vi "Calculate Timing Characteristics.vi"(10 "Engine Clock Rate (MHz)":i32=120000000 format="%.0p", 11 "SPI Signals":T2) -> (3 "Timing Characteristics":T1)   [LabVIEW 2014]
uses:
  Controls/Digital Data.ctl
  Controls/Timing Characteristics.ctl
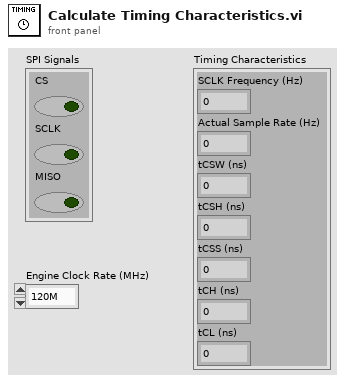
[diagram p1: front panel]
types:
  T1 = typedef "Timing Characteristics.ctl" = cluster{"SCLK Frequency (Hz)":dbl, "Actual Sample Rate (Hz)":dbl, "tCSW (ns)":dbl, "tCSH (ns)":dbl, "tCSS (ns)":dbl, "tCH (ns)":dbl, "tCL (ns)":dbl}
  T2 = typedef "Digital Data.ctl" = cluster{"CS":bool, "SCLK":bool, "MISO":bool}
  T3 = enum16{"A Rising, A Rising", "A Rising, A Falling", "A Falling, A Rising", "A Falling, A Falling", "A Rising, B Rising", "A Rising, B Falling", "A Falling, B Rising", "A Falling, B Falling"}
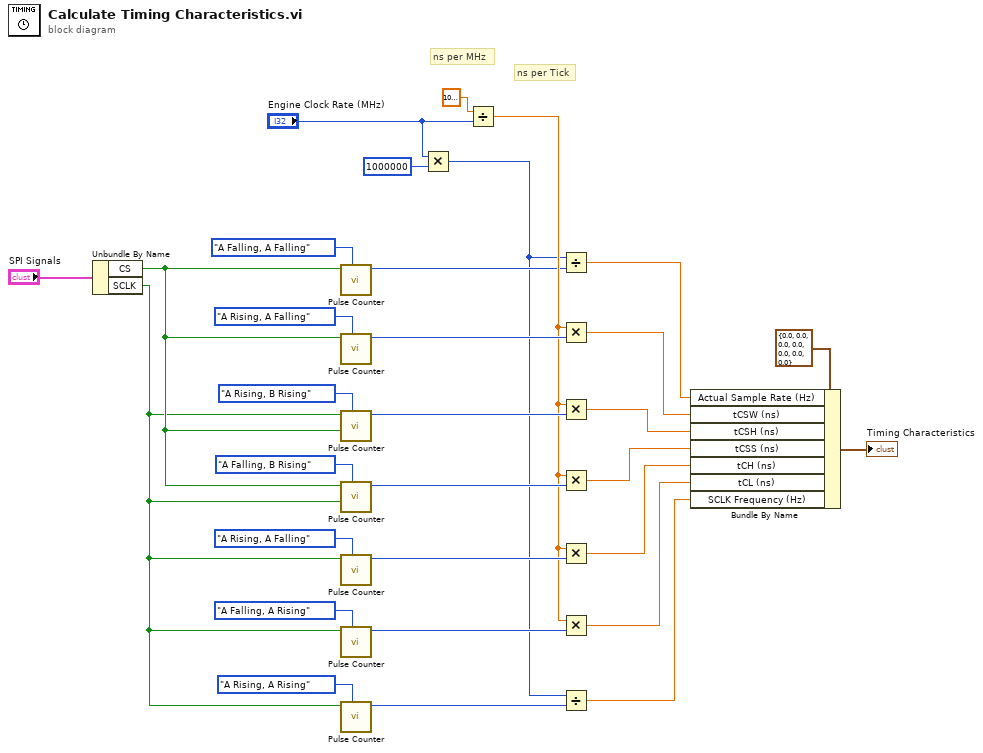
[diagram p0: block diagram]
diagram:
  # "ns per Tick"
  # "ns per MHz"
  n1 = Unbundle By Name("SPI Signals") -> ("CS"=w20:bool, "SCLK"=w14:bool)
  n2 = call "Pulse Counter.vi"("Interval"=T3."A Falling, A Falling", "A"=w20) -> ("Count"=w10:i32)  [unwired: 9 in]
  n3 = call "Pulse Counter.vi"("Interval"=T3."A Rising, A Falling", "A"=w20) -> ("Count"=w19:i32)  [unwired: 9 in]
  n4 = call "Pulse Counter.vi"("Interval"=T3."A Rising, B Rising", "B"=w20, "A"=w14) -> ("Count"=w18:i32)  [unwired: 8 in]
  n5 = call "Pulse Counter.vi"("Interval"=T3."A Falling, B Rising", "B"=w14, "A"=w20) -> ("Count"=w17:i32)  [unwired: 8 in]
  n6 = call "Pulse Counter.vi"("Interval"=T3."A Rising, A Falling", "A"=w14) -> ("Count"=w13:i32)  [unwired: 9 in]
  n7 = call "Pulse Counter.vi"("Interval"=T3."A Falling, A Rising", "A"=w14) -> ("Count"=w12:i32)  [unwired: 9 in]
  n8 = call "Pulse Counter.vi"("Interval"=T3."A Rising, A Rising", "A"=w14) -> ("Count"=w5:i32)  [unwired: 9 in]
  n9 = Multiply(x="Engine Clock Rate (MHz)", y=1000000) -> (x*y=w4:i32)
  n10 = Divide(x=1000.0, y="Engine Clock Rate (MHz)") -> (x/y=w11:dbl)
  n11 = Divide(x=w4, y=w10) -> (x/y=w3:dbl)
  n12 = Multiply(x=w11, y=w19) -> (x*y=w9:dbl)
  n13 = Multiply(x=w11, y=w18) -> (x*y=w8:dbl)
  n14 = Multiply(x=w11, y=w17) -> (x*y=w7:dbl)
  n15 = Multiply(x=w11, y=w13) -> (x*y=w6:dbl)
  n16 = Multiply(x=w11, y=w12) -> (x*y=w2:dbl)
  n17 = Divide(x=w4, y=w5) -> (x/y=w1:dbl)
  n18 = Bundle By Name(cluster=T1 {"SCLK Frequency (Hz)"=0.0, "Actual Sample Rate (Hz)"=0.0, "tCSW (ns)"=0.0, "tCSH (ns)"=0.0, "tCSS (ns)"=0.0, "tCH (ns)"=0.0, "tCL (ns)"=0.0} ("input cluster"), "Actual Sample Rate (Hz)"=w3, "tCSW (ns)"=w9, "tCSH (ns)"=w8, "tCSS (ns)"=w7, "tCH (ns)"=w6, "tCL (ns)"=w2, "SCLK Frequency (Hz)"=w1) -> (→"Timing Characteristics":T1)
